vi "Ejercicio 1.1 y 1.2.vi"() -> ()   [LabVIEW 2020]
panel:
  out "Gauge":dbl(knob) scale=0.0..10.0
  in  "FOCO LED":bool
  out "Nivel de agua":dbl(slide) scale=0.0..10.0
  out "Termostato":dbl(slide) scale=0.0..100.0
  out "String 2":string
  in  "OK Button":bool
  in  "String":string
  in  "stop":bool
  out "LED":bool
  in  "Potencia del ventilador":dbl(knob) scale=0.0..10.0
  in  "Termostato":dbl
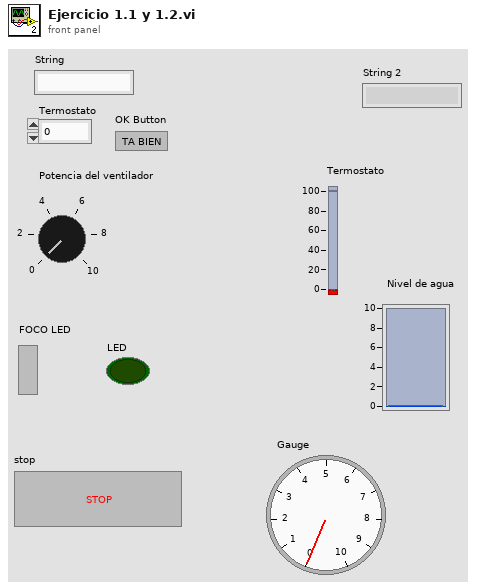
[diagram p1: front panel]
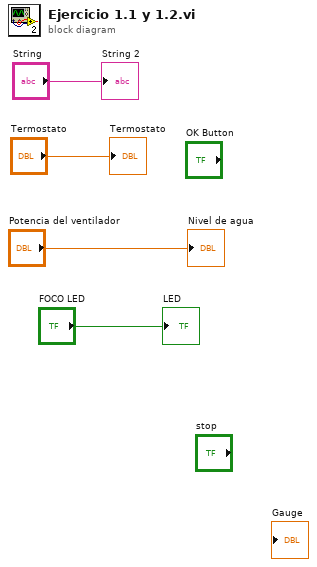
[diagram p0: block diagram]
diagram:
  "LED" <- "FOCO LED"
  "String 2" <- "String"
  "Termostato" <- "Termostato"
  "Nivel de agua" <- "Potencia del ventilador"
